vi "cosmetic ui.vi"(10 "EVENT":refnum<user-event>, 11 "DVR":refnum<data-value>) -> ()   [LabVIEW 2013, in "cosmetic changes.lvclass"]
uses:
  cosmetic changes.lvclass
  VI modification.lvclass
  cosmetic changes.lvclass/cosmetic changes.ctl
  Read don't grow FP.vi
  Read move FP and BD.vi
  Read x (800).vi
  Read y (600).vi
panel:
  in  "don't grow FP (T)":bool=TRUE
  in  "y (600)":i16=600
  in  "x (800)":i16=800
  in  "move FP and BD (T)":bool=TRUE
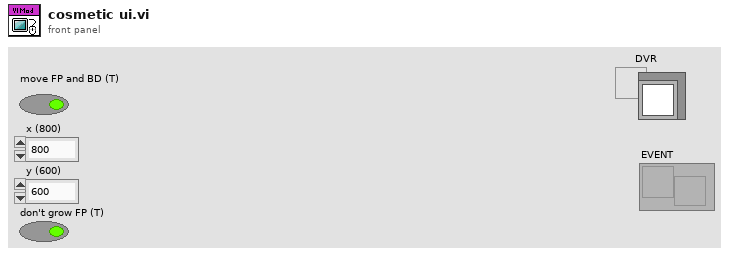
[diagram p1: front panel]
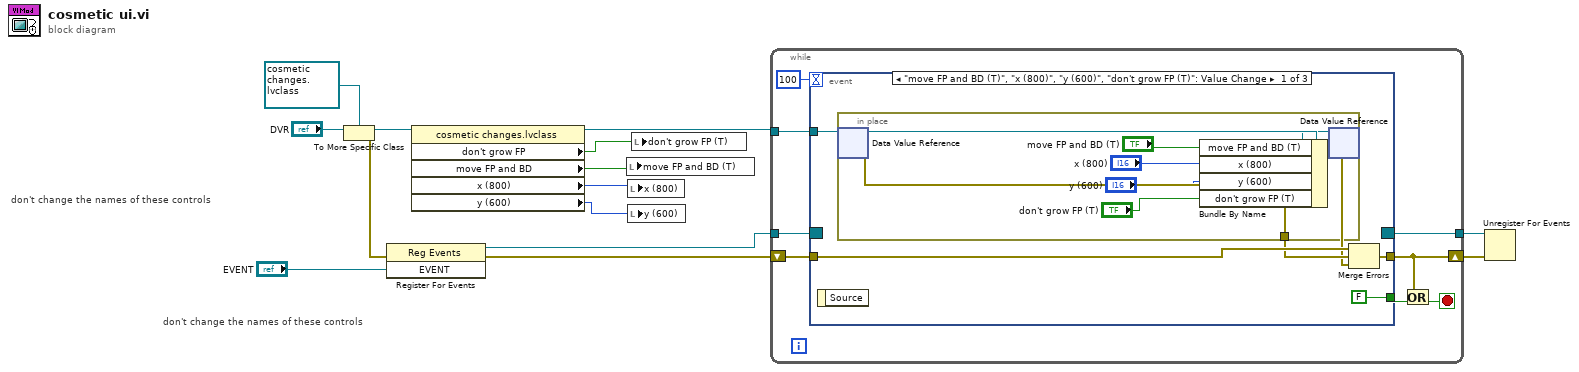
[diagram p0: block diagram]
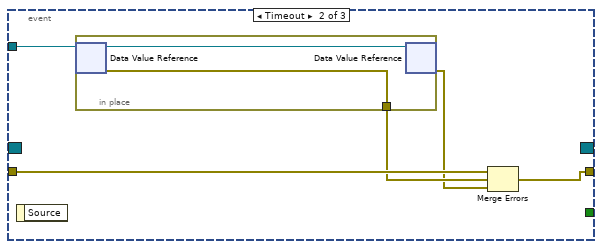
[diagram p2: hidden frame]
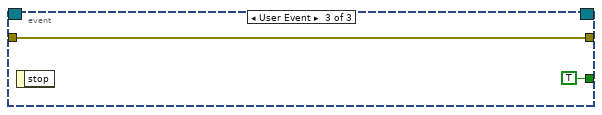
[diagram p3: hidden frame]
diagram:
  # "don't change the names of these controls"
  # "don't change the names of these controls"
  n1 = To More Specific Class(target class=refnum<data-value> refnum, reference="DVR") -> (specific class reference=w8:refnum<data-value>, error out=w6:errorcluster)  [unwired: 1 in]
  n2 = register-events(error in=w6, "EVENT") -> (reference out=w12:refnum<event-registration>, error out=w13:errorcluster)  [unwired: 1 in]
  n3 = property class="cosmetic changes.lvclass"(reference=w8) -> (reference out=w5:refnum<data-value>, "don't grow FP"=w1:bool, "move FP and BD"=w3:bool, "x (800)"=w4:i16, "y (600)"=w2:i16)  [unwired: 1 in, 1 out]
  n4 = local write "move FP and BD (T)"(w3) -> ()
  n5 = local write "x (800)"(w4) -> ()
  n6 = local write "y (600)"(w2) -> ()
  n7 = local write "don't grow FP (T)"(w1) -> ()
  n8 = while {
    shift-right: [w15] -> w11
    shift-left: w13 -> [w19]
    tunnel: w12 -> [w22]
    tunnel: [w21] -> w10
    tunnel: w5 -> [w18]
    stop <- w16 stop-if-true
    n9 = event shown="[0] \"move FP and BD (T)\", \"x (800)\", \"y (600)\", \"don't grow FP (T)\": Value Change" {
      selector: w22 -> [_ _ _]
      dyn-events: [_ _ _] -> w21
      timeout: 100 -> [_ _ _]
      tunnel: [FALSE _ TRUE] -> w20
      tunnel: [w26 w38 w44] -> w15
      tunnel: w19 -> [w28 w39 w44]
      tunnel: w18 -> [w27 w40 _]
      event "move FP and BD (T)", "x (800)", "y (600)", "don't grow FP (T)": Value Change {
        n10 = event-data() -> ()  [unwired: 1 in, 1 out]
        n11 = in-place {
          in-place-border: [w33] -> w24
          n12 = in-place-dvr #1(w27) -> (w35:refnum<class "cosmetic changes.lvclass">, w33:errorcluster)
          n13 = Bundle By Name(cluster=w35, "move FP and BD (T)"="move FP and BD (T)", "x (800)"="x (800)", "y (600)"="y (600)", "don't grow FP (T)"="don't grow FP (T)") -> (w34:refnum<class "cosmetic changes.lvclass">)
          n14 = in-place-dvr #1(w34) -> (w23:errorcluster)  [unwired: 1 out]
        }
        n15 = Merge Errors(w28, w24, w23) -> (w26:errorcluster)
      }
      event Timeout {
        n16 = event-data() -> ()  [unwired: 1 in, 1 out]
        n17 = in-place {
          in-place-border: [w41] -> w37
          n18 = in-place-dvr #2(w40) -> (w42:refnum<class "cosmetic changes.lvclass">, w41:errorcluster)
          n19 = in-place-dvr #2(w42) -> (w36:errorcluster)  [unwired: 1 out]
        }
        n20 = Merge Errors(w39, w37, w36) -> (w38:errorcluster)
      }
      event User Event {
        n21 = event-data() -> ()  [unwired: 1 in, 1 out]
      }
    }
    n22 = Or(x=w15, y=w20) -> (x .or. y?=w16:bool)
  }
  n23 = Unregister For Events(event registration refnum=w10, error in=w11) -> ()  [unwired: 1 out]
